vi "IsOverlap.vi"(4 "TheirSize":T1, 5 "YourSize":T1, 6 "TheirPosition":T1, 7 "YourPosition":T2, 8 "error in (no error)":errorcluster, 11 "VelocityIn":T2) -> (0 "error out":errorcluster, 2 "Collision?":bool, 3 "Velocity out":T2)   [LabVIEW 2019, in "RT_Game.lvlib" / "PongBall.lvclass"]
uses:
  PongBall.lvclass
  Game/Coordinate.ctl
  Velocity.ctl
  Game/Game.lvclass
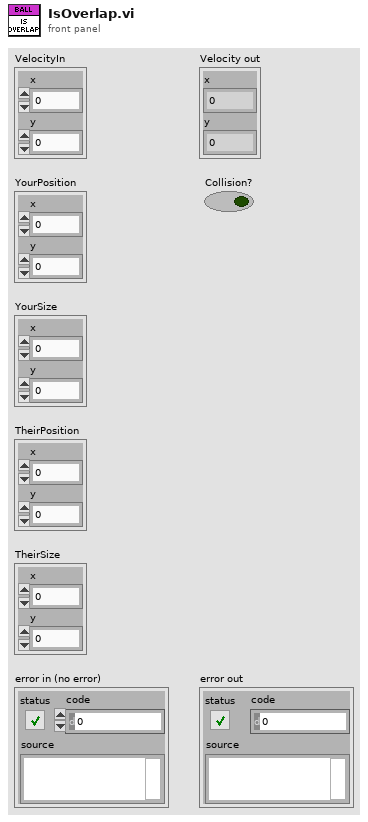
[diagram p1: front panel]
types:
  T1 = typedef "RT_Game.lvlib/Game.lvclass/Coordinate.ctl" = cluster{"x":dbl, "y":dbl}
  T2 = typedef "Velocity.ctl" = cluster{"x":dbl, "y":dbl}
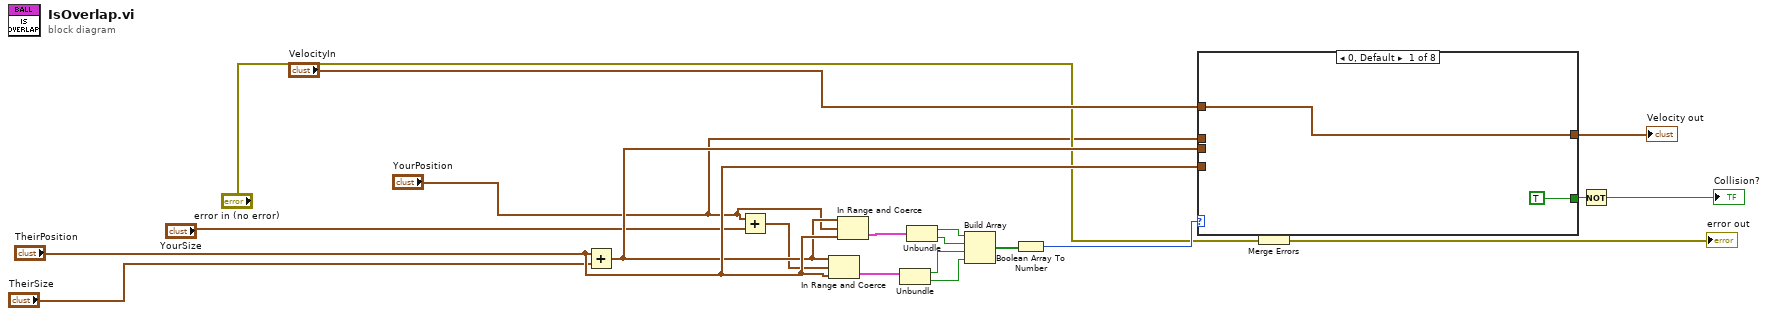
[diagram p0: block diagram]
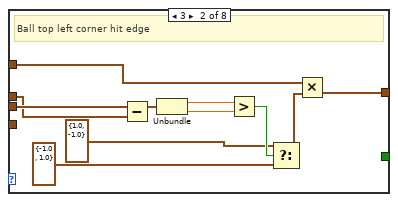
[diagram p2: hidden frame]
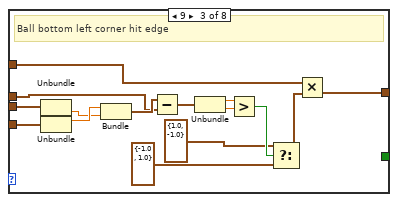
[diagram p3: hidden frame]
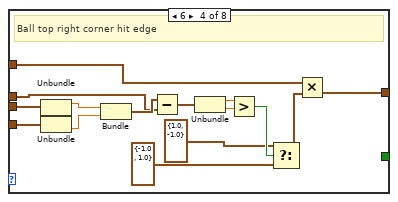
[diagram p4: hidden frame]
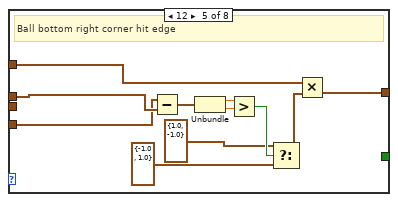
[diagram p5: hidden frame]
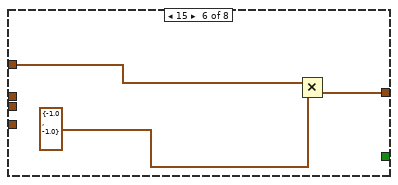
[diagram p6: hidden frame]
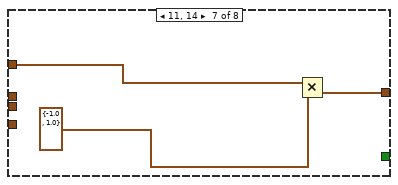
[diagram p7: hidden frame]
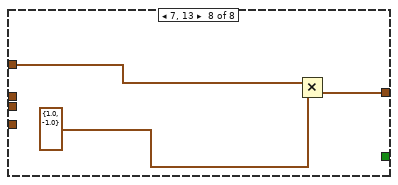
[diagram p8: hidden frame]
diagram:
  n1 = Add(x="TheirPosition", y="TheirSize") -> (x+y=w16:T1)
  n2 = Add(x="YourPosition", y="YourSize") -> (x+y=w4:T2)
  n3 = In Range and Coerce(upper limit=w16, x=w4, lower limit="TheirPosition") -> (In Range?=w7:cluster{"x":bool, "y":bool})  [unwired: 1 out]
  n4 = In Range and Coerce(upper limit=w16, x="YourPosition", lower limit="TheirPosition") -> (In Range?=w6:cluster{"x":bool, "y":bool})  [unwired: 1 out]
  n5 = Unbundle(w7) -> ("x"=w10:bool, "y"=w11:bool)
  n6 = Unbundle(w6) -> ("x"=w8:bool, "y"=w9:bool)
  n7 = Build Array(w8, w9, w10, w11) -> (w12:bool[])
  n8 = Boolean Array To Number(Boolean array=w12) -> (number=w13:u32)
  n9 = case shown="0, Default" w13 {
    tunnel: "VelocityIn" -> [w22 w33 w48 w63 w74 w77 w80 w83]
    tunnel: [w22 w32 w47 w62 w73 w76 w79 w82] -> w15
    tunnel: w16 -> [_ w31 w41 w56 _ _ _ _]
    tunnel: "YourPosition" -> [_ w27 w37 w54 w68 _ _ _]
    tunnel: "TheirPosition" -> [_ _ w42 w57 w64 _ _ _]
    tunnel: [TRUE _ _ _ _ _ _ _] -> w18
    frame 0, Default {
    }
    frame 3 {
      # "Ball top left corner hit edge"
      n10 = Subtract(x=w31, y=w27) -> (x-y=w28:T1)
      n11 = Unbundle(w28) -> ("x"=w30:dbl, "y"=w29:dbl)
      n12 = Greater?(x=w30, y=w29) -> (0:w24:bool)
      n13 = Select(t=T2 {"x"=1.0, "y"=-1.0}, s=w24, f=T2 {"x"=-1.0, "y"=1.0} ("x")) -> (s? t:f=w26:T2)
      n14 = Multiply(x=w33, y=w26) -> (x*y=w32:T2)
    }
    frame 9 {
      # "Ball bottom left corner hit edge"
      n15 = Unbundle(w41) -> ("y"=w39:dbl)  [unwired: 1 out]
      n16 = Unbundle(w42) -> ("x"=w40:dbl)  [unwired: 1 out]
      n17 = Bundle("x"=w40, "y"=w39) -> (w38:cluster{"x":dbl, "y":dbl})  [unwired: 1 in]
      n18 = Subtract(x=w38, y=w37) -> (x-y=w36:T2)
      n19 = Unbundle(w36) -> ("x"=w35:dbl, "y"=w34:dbl)
      n20 = Greater?(x=w35, y=w34) -> (0:w44:bool)
      n21 = Select(t=T2 {"x"=1.0, "y"=-1.0}, s=w44, f=T2 {"x"=-1.0, "y"=1.0} ("x")) -> (s? t:f=w46:T2)
      n22 = Multiply(x=w48, y=w46) -> (x*y=w47:T2)
    }
    frame 6 {
      # "Ball top right corner hit edge"
      n23 = Unbundle(w56) -> ("x"=w50:dbl)  [unwired: 1 out]
      n24 = Unbundle(w57) -> ("y"=w49:dbl)  [unwired: 1 out]
      n25 = Bundle("x"=w50, "y"=w49) -> (w55:cluster{"x":dbl, "y":dbl})  [unwired: 1 in]
      n26 = Subtract(x=w55, y=w54) -> (x-y=w53:T2)
      n27 = Unbundle(w53) -> ("x"=w52:dbl, "y"=w51:dbl)
      n28 = Greater?(x=w52, y=w51) -> (0:w59:bool)
      n29 = Select(t=T2 {"x"=1.0, "y"=-1.0}, s=w59, f=T2 {"x"=-1.0, "y"=1.0} ("x")) -> (s? t:f=w61:T2)
      n30 = Multiply(x=w63, y=w61) -> (x*y=w62:T2)
    }
    frame 12 {
      # "Ball bottom right corner hit edge"
      n31 = Subtract(x=w64, y=w68) -> (x-y=w67:T1)
      n32 = Unbundle(w67) -> ("x"=w66:dbl, "y"=w65:dbl)
      n33 = Greater?(x=w66, y=w65) -> (0:w70:bool)
      n34 = Select(t=T2 {"x"=1.0, "y"=-1.0}, s=w70, f=T2 {"x"=-1.0, "y"=1.0} ("x")) -> (s? t:f=w72:T2)
      n35 = Multiply(x=w74, y=w72) -> (x*y=w73:T2)
    }
    frame 15 {
      n36 = Multiply(x=w77, y=T2 {"x"=-1.0, "y"=-1.0} ("x")) -> (x*y=w76:T2)
    }
    frame 11, 14 {
      n37 = Multiply(x=w80, y=T2 {"x"=-1.0, "y"=1.0} ("x")) -> (x*y=w79:T2)
    }
    frame 7, 13 {
      n38 = Multiply(x=w83, y=T2 {"x"=1.0, "y"=-1.0} ("x")) -> (x*y=w82:T2)
    }
  }
  "Velocity out" <- w15
  n39 = Merge Errors("error in (no error)") -> (→"error out":errorcluster)
  n40 = Not(x=w18) -> (.not. x?=→"Collision?":bool)
